vi "Pre Launch Init.vi"(11 "Vacuum in":refnum<class "Vacuum.lvclass">) -> (0 "error out":errorcluster, 3 "Vacuum out":refnum<class "Vacuum.lvclass">)   [LabVIEW 2015, in "AMS UI.lvlib" / "Vacuum.lvclass"]
doc: "(<B>Filename</B>: Actor Framework.lvlib:Actor.lvclass:Pre Launch Init.vi)\n\nDefines behavior that occurs after the Launch Actor method is invoked but before the actor's Actor Core method begins running.\n\nThe Pre Launch Init method is guaranteed to finish before the Launch Actor method returns to its caller and before the actor itself receives any messages. Any references that the Pre Launch Init method obtains are guaranteed to have the same lifetime as the actor itself. Any errors that the Pre Launch Init method returns will abort the launch.\n\nBy default, this method does nothing. A descendant class may override it to define behavior."
uses:
  Vacuum.lvclass
  eActor Messages/Timeout Msg/Timeout Msg.lvclass
  <vilib>/ActorFramework/Message Enqueuer/Message Priority.ctl
  AMS Gas Actor/AMS Gas Actor.lvclass
  <vilib>/ActorFramework/Message Enqueuer/Message Enqueuer.lvclass
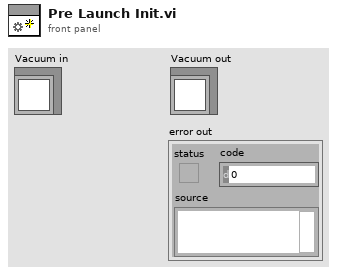
[diagram p1: front panel]
types:
  T1 = typedef "Actor Framework.lvlib/Message Enqueuer.lvclass/Message Priority.ctl" = enum16{"Low", "Normal", "High"}
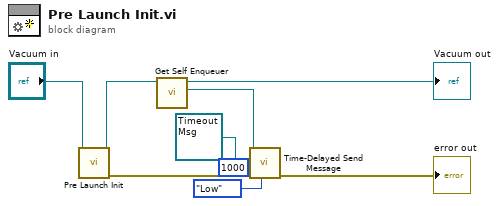
[diagram p0: block diagram]
diagram:
  n1 = call-parent "Pre Launch Init.vi"("eActor in"="Vacuum in") -> ("error out"=w6:errorcluster, "eActor out"=w8:refnum<class "Vacuum.lvclass">)  [unwired: 9 in]
  n2 = call-dynamic "Get Self Enqueuer.vi"("eActor in"=w8) -> ("Actor Framework:Message Enqueuer"=w4:refnum<class "Message Enqueuer.lvclass">, "eActor out"=→"Vacuum out":refnum<class "Vacuum.lvclass">)  [unwired: 9 in]
  n3 = call <vilib>:"Time-Delayed Send Message.vi"("Message Priority (Normal)"=Message_Priority."Low", "error in (no error)"=w6, "Milliseconds To Wait"=1000, "Message"=refnum<class "Timeout Msg.lvclass"> refnum ("Timeout Msg.lvclass"), "Message Enqueuer"=w4) -> ("error out"=→"error out":errorcluster)  [unwired: 5 in, 1 out]
